vi "GetCtlRef_Core.vi"(8 "error in (no error)":errorcluster, 10 "CtlName In":string, 11 "CtlReferences in":refnum<class "CtlReferences.lvclass">) -> (0 "error out":errorcluster, 1 "Ctl Refnum":refnum<vi>, 2 "CtlName out":string, 3 "CtlReferences out":refnum<class "CtlReferences.lvclass">, 4 "Found":bool)   [LabVIEW 2020, in "CtlReferences.lvlib" / "CtlReferences.lvclass"]
uses:
  CtlReferences.lvclass
  CtlReferences.lvclass/CtlReferences.ctl
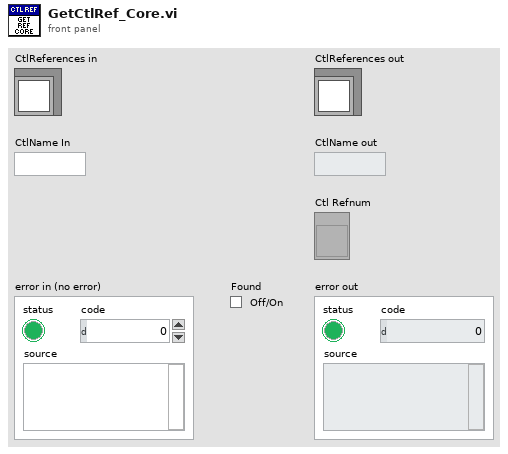
[diagram p1: front panel]
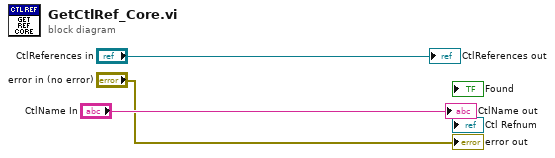
[diagram p0: block diagram]
diagram:
  "CtlName out" <- "CtlName In"
  "CtlReferences out" <- "CtlReferences in"
  "error out" <- "error in (no error)"
